vi "Digital Pulse Acquire_RPM.vi"() -> ()   [LabVIEW 2019]
uses:
  <vilib>/Utility/error.llb/DialogType.ctl
  <vilib>/DAQmx/create/channels.llb/DAQmx Create Channel (CO-Pulse Generation-Time).vi
  <vilib>/DAQmx/configure/timing.llb/DAQmx Timing (Implicit).vi
  <resource>/objmgr/daqmx.rc
panel:
  out "Delay Time":dbl
  out "Frequency":dbl
  out "Period":dbl
  in  "RPM":dbl
  out "CO.CtrTimebaseRate 2":dbl format="%#_6f"
  out "CO.CtrTimebaseSrc":tag
  out "CO.Pulse.Term":tag
  out "CO.Pulse.HighTime":dbl
  out "CO.Pulse.LowTime":dbl
  out "SampQuant.SampPerChan":dbl
  in  "Counter to Output with":tag="Dev1/ctr0"
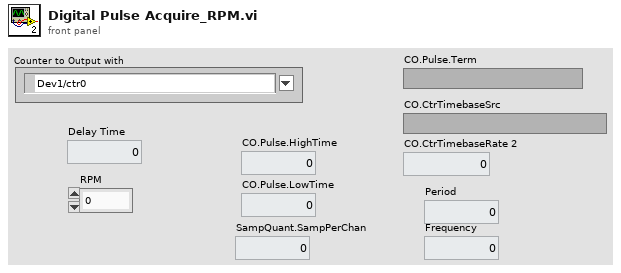
[diagram p1: front panel]
types:
  T1 = typedef "DialogType.ctl" = u16
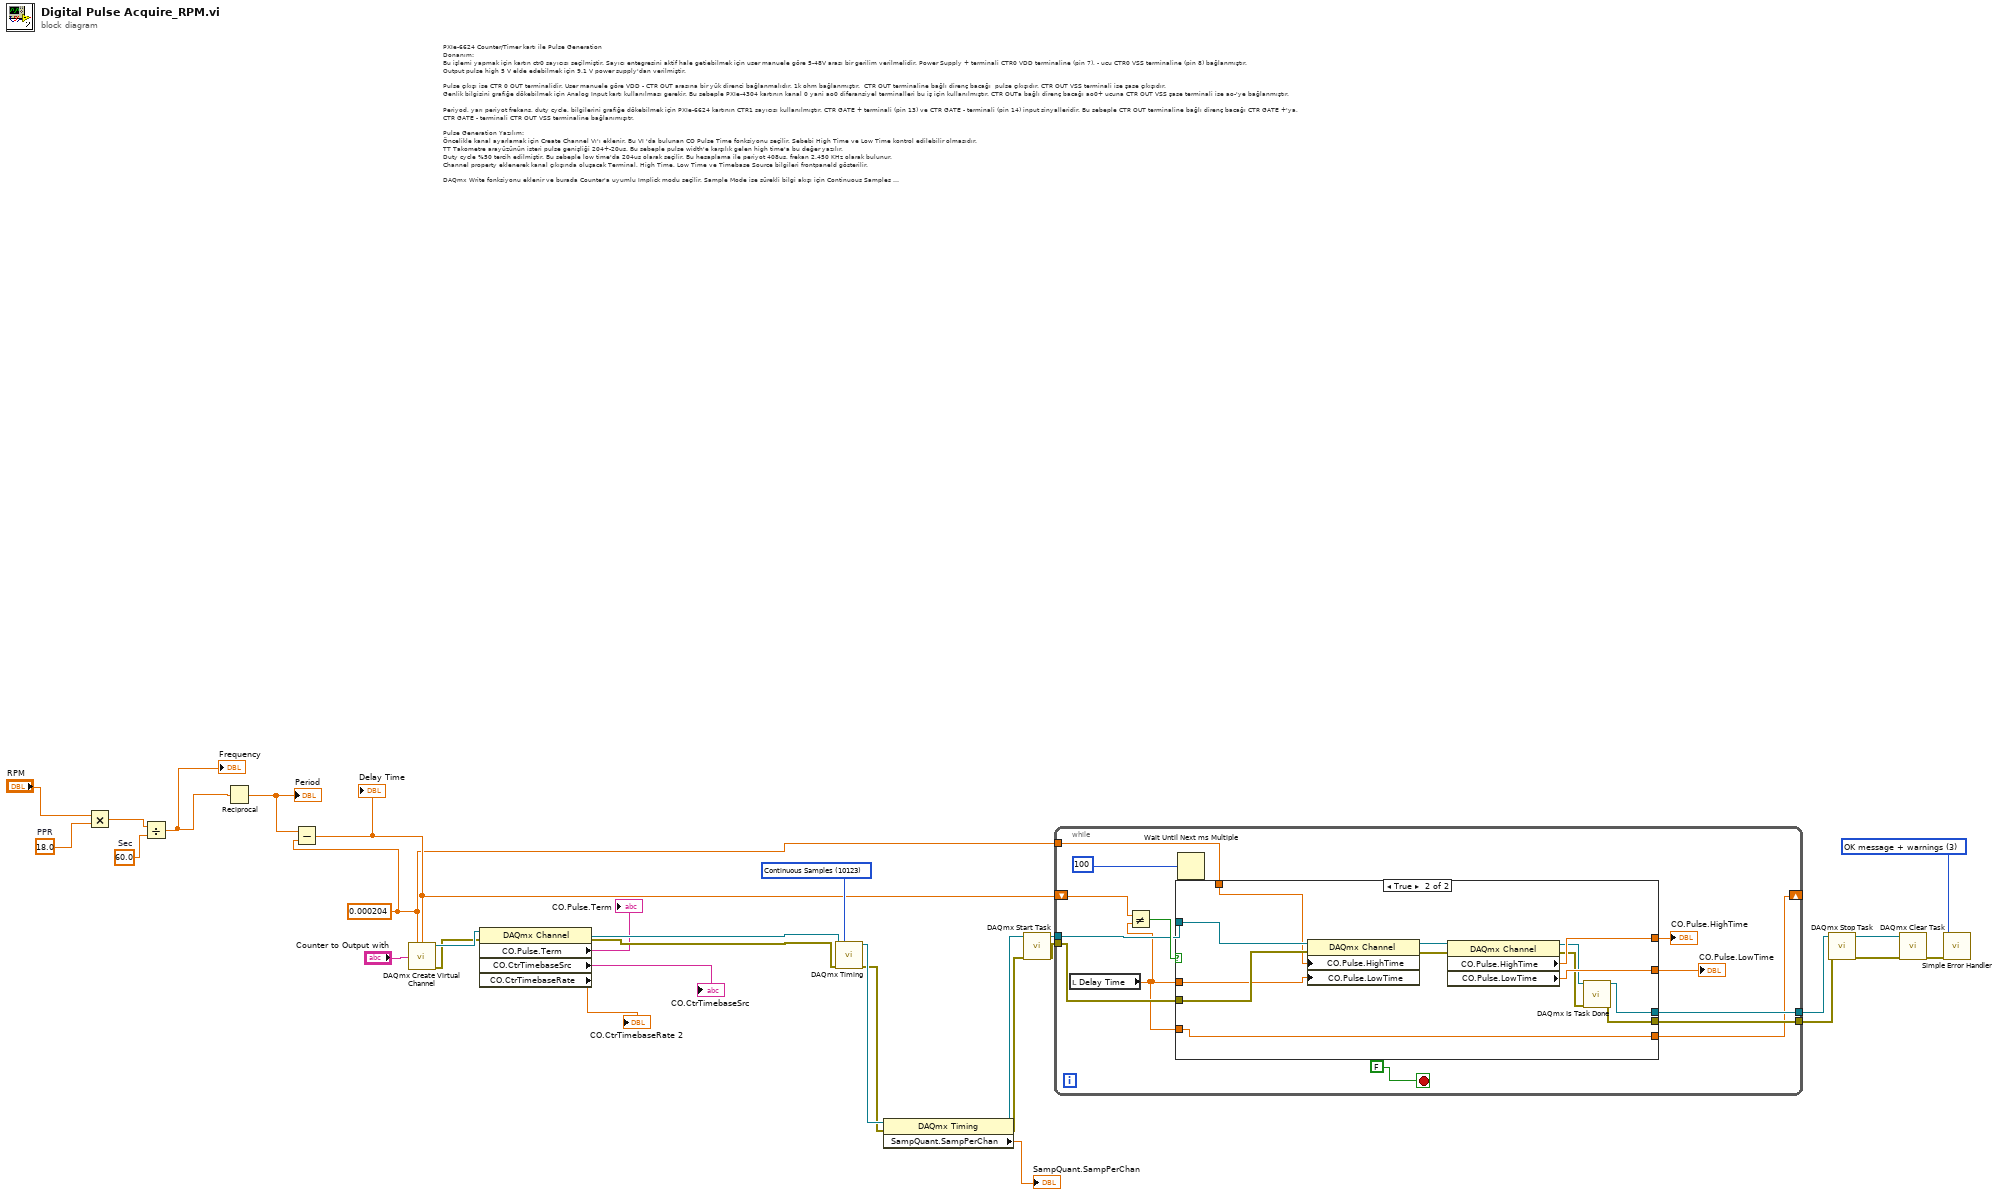
[diagram p0: block diagram]
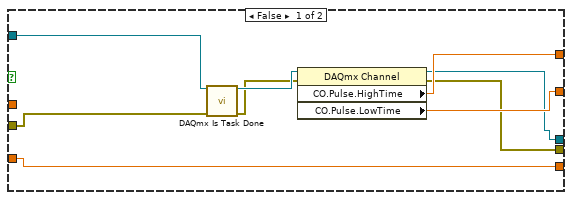
[diagram p2: hidden frame]
diagram:
  w3 = 18.0  # PPR
  w7 = 60.0  # Sec
  w1 = 0.000204 ("high time")
  w24 = T1 3 items=["no dialog", "OK message", "continue or stop message", "OK message + warnings", "continue/stop + warnings"] ("type of dialog (OK msg:1)")
  w27 = 10123 items=["Finite Samples"=10178, "Continuous Samples"=10123, "Hardware Timed Single Point"=12522] ("sample mode")
  # "PXIe-6624 Counter/Timer kartı ile Pulse Generation\nDonanım:\nBu işlemi yapmak için kartın ctr0 sayıcısı seçilmiştir. Sayıcı entegresini aktif hale getiebilmek için user manuele göre 5-48V arası bir gerilim verilmelidir. Power Supply + terminali CTR0 VDD terminaline (pin 7), - ucu CTR0 VSS terminaline (pin 8) bağlanmıştır. \nOutput pulse high 5 V elde edebilmek için 9.1 V power supply'dan verilmiştir. \n\nPulse çıkışı ise CTR 0 OUT terminalidir. User manuele göre VDD - CTR OUT arasına bir yük direnci bağlanmalıdır. 1k ohm bağlanmıştır.  CTR OUT terminaline bağlı direnç bacağı  pulse çıkışıdır. CTR OUT VSS terminali ise şase çıkışıdır.\nGenlik bilgisini grafiğe dökebilmek için Analog Input kartı kullanılması gerekir. Bu sebeple PXIe-4304 kartının kanal 0 yani ao0 diferansiyel terminalleri bu iş için kullanılmıştır. CTR OUTa bağlı direnç bacağı ao0+ ucuna CTR OUT VSS şase terminali ise ao-'ye bağlanmıştır.\n\nPeriyod, yarı periyot frekans, duty cycle, bilgilerini grafiğe dökebilmek için PXIe-6624 kartının CTR1 sayıcısı kullanılmıştır. CTR GATE + terminali (pin 13) ve CTR GATE - terminali (pin 14) input sinyalleridir. Bu sebeple CTR OUT terminaline bağlı direnç bacağı CTR GATE +'ya,\nCTR GATE - terminali CTR OUT VSS terminaline bağlanımışıtr. \n\nPulse Generation Yazılım:\nÖncelikle kanal ayarlamak için Create Channel Vı'ı eklenir. Bu VI 'da bulunan CO Pulse Time fonksiyonu seçilir. Sebebi High Time ve Low Time kontrol edilebilir olmasıdır. \nTT Takometre arayüzünün isteri pulse genişliği 204+-20us. Bu sebeple pulse width'e karşılık gelen high time'a bu değer yazılır. \nDuty cycle %50 tercih edilmiştir. Bu sebeple low time'da 204us olarak seçilir. Bu hesaplama ile periyot 408us, frekan 2.450 KHz olarak bulunur.\nChannel property eklenerek kanal çıkışında oluşacak Terminal, High Time, Low Time ve Timebase Source bilgileri frontpaneld gösterilir.\n\nDAQmx Write fonksiyonu eklenir ve burada Counter'a uyumlu Implick modu seçilir. Sample Mode ise sürekli bilgi akışı için Continuous Samples seçilir.\nGörevi başlatmak için Start VI'ı eklenir.\nStop btonuna basana kadar dönecek DAQmx is Task Done Vı'ı ile pulse üretimi gerçekleştirilir."
  n1 = Multiply(x="RPM", y=w3) -> (x*y=w8:dbl)
  n2 = Divide(x=w8, y=w7) -> (x/y=w6:dbl)
  "Frequency" <- w6
  n3 = Reciprocal(x=w6) -> (1/x=w4:dbl)
  "Period" <- w4
  n4 = Subtract(x=w4, y=w1) -> (x-y=w2:dbl)
  "Delay Time" <- w2
  n5 = call-poly <vilib>:"DAQmx Create Virtual Channel.vi"("high time"=w1, "low time"=w2, "counter"="Counter to Output with") -> ("task out"=w13:refnum<k21>, "error out"=w12:errorcluster)  [unwired: 11 in]
  n6 = property class="DAQmx Channel"(reference=w13, error in=w12) -> (reference out=w28:refnum<k21>, error out=w29:errorcluster, "CO.Pulse.Term"=→"CO.Pulse.Term":tag, "CO.CtrTimebaseSrc"=→"CO.CtrTimebaseSrc":tag, "CO.CtrTimebaseRate"=→"CO.CtrTimebaseRate 2":dbl)
  n7 = call-poly <vilib>:"DAQmx Timing.vi"("task/channels in"=w28, "sample mode"=w27, "error in"=w29) -> ("task out"=w23:refnum<k21>, "error out"=w22:errorcluster)  [unwired: 11 in]
  n8 = property class="DAQmx Timing"(reference=w23, error in=w22) -> (reference out=w21:refnum<k21>, error out=w20:errorcluster, "SampQuant.SampPerChan"=→"SampQuant.SampPerChan":dbl)
  n9 = call <vilib>:"DAQmx Start Task.vi"("task/channels in"=w21, "error in"=w20) -> ("task out"=w26:refnum<k21>, "error out"=w18:errorcluster)  [unwired: 12 in]
  n10 = while {
    tunnel: w18 -> [w39]
    tunnel: w26 -> [w40]
    shift-right: [w32] -> _
    shift-left: w2 -> [w33]
    tunnel: w1 -> [w38]
    tunnel: [w37] -> w15
    tunnel: [w36] -> w14
    stop <- FALSE stop-if-true
    n11 = local read "Delay Time"() -> (w31:dbl)
    n12 = Not Equal?(x=w33, y=w31) -> (x != y?=w41:bool)
    n13 = case shown="True" w41 {
      tunnel: w40 -> [w52 w65]
      tunnel: w39 -> [w51 w64]
      tunnel: w38 -> [_ w61]
      tunnel: [w46 w63] -> w37
      tunnel: [w45 w62] -> w36
      tunnel: [w48 w58] -> w35
      tunnel: [w47 w57] -> w34
      tunnel: w31 -> [w44 w53]
      tunnel: [w44 w53] -> w32
      tunnel: w31 -> [_ w54]
      frame False {
        n14 = call <vilib>:"DAQmx Is Task Done.vi"("task/channels in"=w52, "error in"=w51) -> ("task out"=w50:refnum<k21>, "error out"=w49:errorcluster)  [unwired: 11 in, 1 out]
        n15 = property class="DAQmx Channel"(reference=w50, error in=w49) -> (reference out=w46:refnum<k21>, error out=w45:errorcluster, "CO.Pulse.HighTime"=w48:dbl, "CO.Pulse.LowTime"=w47:dbl)
      }
      frame True {
        n16 = property class="DAQmx Channel"(reference=w65, error in=w64, "CO.Pulse.HighTime"=w61, "CO.Pulse.LowTime"=w54) -> (reference out=w60:refnum<k21>, error out=w59:errorcluster)
        n17 = property class="DAQmx Channel"(reference=w60, error in=w59) -> (reference out=w56:refnum<k21>, error out=w55:errorcluster, "CO.Pulse.HighTime"=w58:dbl, "CO.Pulse.LowTime"=w57:dbl)
        n18 = call <vilib>:"DAQmx Is Task Done.vi"("task/channels in"=w56, "error in"=w55) -> ("task out"=w63:refnum<k21>, "error out"=w62:errorcluster)  [unwired: 11 in, 1 out]
      }
    }
    "CO.Pulse.HighTime" <- w35
    "CO.Pulse.LowTime" <- w34
    n19 = Wait Until Next ms Multiple(millisecond multiple=100) -> ()  [unwired: 1 out]
  }
  n20 = call <vilib>:"DAQmx Stop Task.vi"("task/channels in"=w15, "error in"=w14) -> ("task out"=w17:refnum<k21>, "error out"=w16:errorcluster)  [unwired: 12 in]
  n21 = call <vilib>:"DAQmx Clear Task.vi"("task in"=w17, "error in"=w16) -> ("error out"=w25:errorcluster)  [unwired: 13 in]
  n22 = call <vilib>:"Simple Error Handler.vi"("type of dialog (OK msg:1)"=w24, "error in (no error)"=w25) -> ()  [unwired: 3 in, 5 out]
